vi "Set_TargetFile_Name.vi"(7 "Target OS":T1(ring), 8 "error in (no error)":errorcluster, 9 "Target file type":T2, 10 "Target file name":string, 11 "AB_DepDLL in":refnum<class "AB_DepDLL.lvclass">) -> (0 "error out":errorcluster, 3 "AB_DepDLL out":refnum<class "AB_DepDLL.lvclass">)   [LabVIEW 2020, in "AB_DepDLL.lvclass"]
uses:
  <vilib>/AppBuilder/AB_Classes/DepDLL/AB_DepDLL.lvclass
  e:/builds/penguin/labview/branches/2020/dev/dist/vi.lib/AppBuilder/AB_Classes/TargetFile/AB_Targetfile.lvclass
  <vilib>/AppBuilder/AB_TargetFileType.ctl
  <resource>/Framework/Providers/Common/provcom_StringGlobals.vi
  <vilib>/AppBuilder/AB_Classes/TargetFile/AB_Targetfile.lvclass
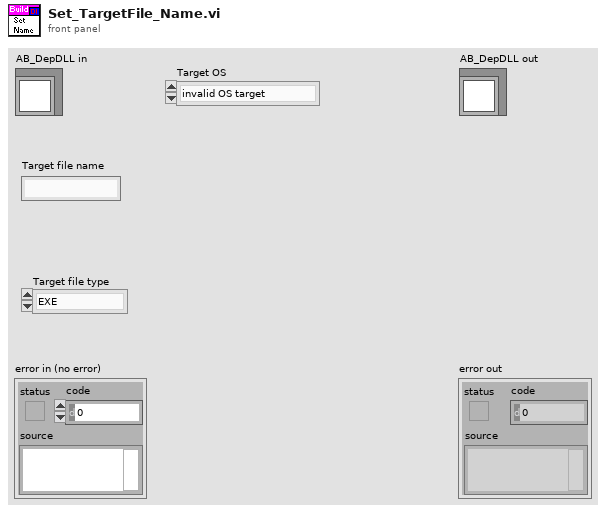
[diagram p1: front panel]
types:
  T1 = enum32{"invalid OS target", "Mac OS", "Windows 3.1", "Windows 95/NT", "Solaris 1", "Solaris 2", "HP-UX", "PowerMAX", "Linux", "Irix", "Rhapsody", "BeOS", "AIX", "OSF1", "VxWorks", "PharLap", "Carbon", "RTX", "Windows x64", "Linux x64", "Mac OS X x64"}
  T2 = typedef "AB_TargetFileType.ctl" = enum16{"EXE", "DLL", "RTEXE"}
  T3 = typedef "AB_Targetfile.ctl" = cluster{"targetfileName":string, "targetfileGUID":string, "enableDebugging":bool, "versionInfo":cluster{"productName":string, "legalCopyright":string, "companyName":string, "internalName":string, "fileDescription":string}, "eng_consolidatedTypeInfo":string, "fastFileFormat":bool, "eng_LEIFBuildData":u32, "versionIndependent":bool}
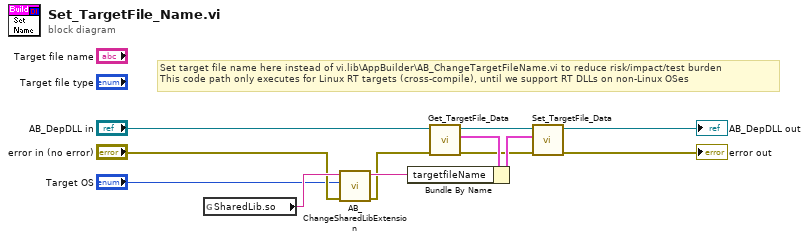
[diagram p0: block diagram]
diagram:
  # "Set target file name here instead of vi.lib\\AppBuilder\\AB_ChangeTargetFileName.vi to reduce risk/impact/test burden\nThis code path only executes for Linux RT targets (cross-compile), until we support RT DLLs on non-Linux OSes"
  n1 = global read "provcom_StringGlobals.vi" "SharedLib.so"() -> (w6:string)
  n2 = call <vilib>:"AB_ChangeSharedLibExtension.vi"("error in (no error)"="error in (no error)", "Target OS"="Target OS", "Target file name"=w6) -> ("error out"=w5:errorcluster, "New target file name"=w9:string)  [unwired: 7 in]
  n3 = call <vilib>:"Get_TargetFile_Data.vi"("error in (no error)"=w5, "AB_Targetfile in"="AB_DepDLL in") -> ("error out"=w4:errorcluster, "data"=w12:T3, "AB_Targetfile out"=w10:refnum<class "AB_DepDLL.lvclass">)  [unwired: 7 in]
  n4 = Bundle By Name(cluster=w12, "targetfileName"=w9) -> (w11:T3)
  n5 = call <vilib>:"Set_TargetFile_Data.vi"("error in (no error)"=w4, "data"=w11, "AB_Targetfile in"=w10) -> ("error out"=→"error out":errorcluster, "AB_Targetfile out"=→"AB_DepDLL out":refnum<class "AB_DepDLL.lvclass">)  [unwired: 7 in]
